vi "MHL Cases.vi"(8 "error in":errorcluster, 11 "Worker Base Class in":refnum<class "Worker Base Class.lvclass">) -> (0 "error out":errorcluster, 3 "Worker Base Class out":refnum<class "Worker Base Class.lvclass">)   [LabVIEW 2017, in "Worker Base Class.lvclass"]
doc: "The base class Message Handling Loop cases of a Worker's QMH."
uses:
  Worker Base Class.lvclass
  C:/Program Files (x86)/National Instruments/LabVIEW 2017/vi.lib/addons/_Workers/Library/Classes/Worker/Worker.lvclass
  <vilib>/addons/_Workers/Library/Classes/Worker/Worker.lvclass/Worker.ctl
  <vilib>/addons/_Workers/Library/Classes/Message/Message.lvclass/Message.ctl
  Initialization Data.ctl
  Response Cases.ctl
  Worker Base Class.lvclass/Worker Base Class.ctl
  rqp_Send message to Caller.ctl
  rqp_Send message to subWorkers.ctl
  <vilib>/addons/_Workers/Library/Classes/Worker/Worker.lvclass
  <vilib>/addons/_Workers/Library/Classes/Message/Message.lvclass
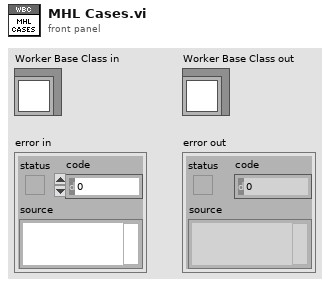
[diagram p1: front panel]
types:
  T1 = typedef "Workers.lvlib/Case Label.ctl" = string
  T2 = typedef "Worker Base Class.lvclass/Initialization Data.ctl" = cluster{"Response Cases":T3}
  T3 = typedef "Worker Base Class.lvclass/Response Cases.ctl" = cluster{"Placeholder - Can be deleted":string}
  T4 = typedef "Worker Base Class.lvclass/rqp_Send message to Caller.ctl" = cluster{"String":string}
  T5 = typedef "Worker Base Class.lvclass/rqp_Send message to subWorkers.ctl" = cluster{"String":string}
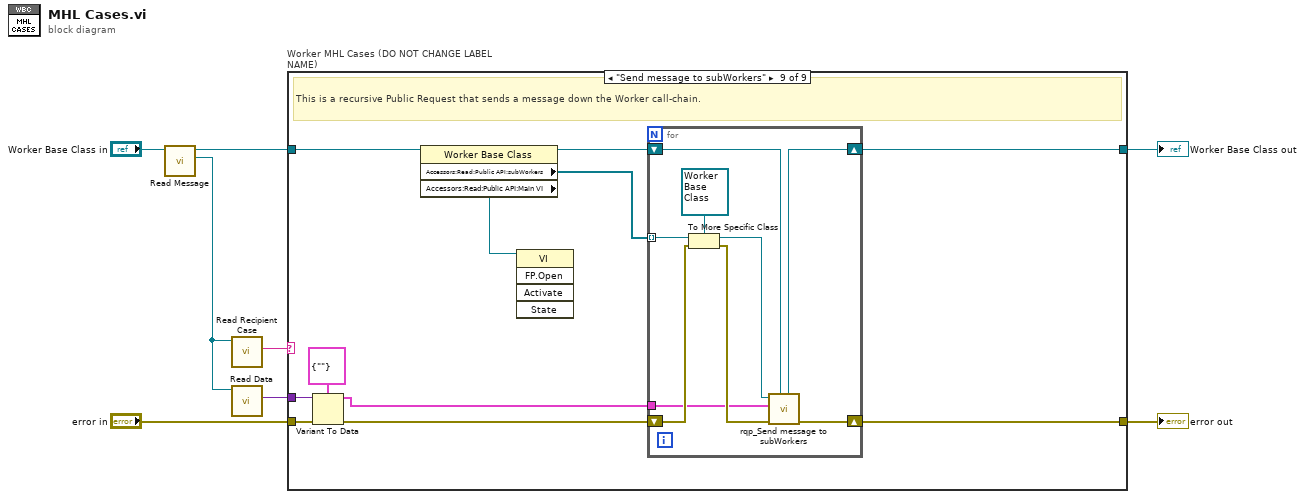
[diagram p0: block diagram]
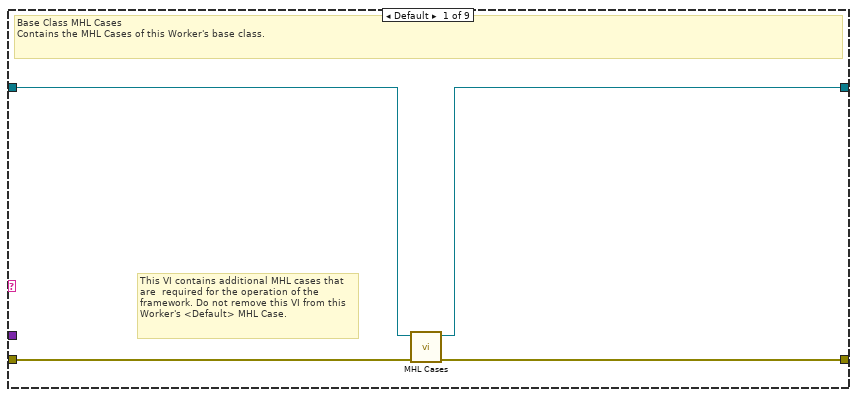
[diagram p2: hidden frame]
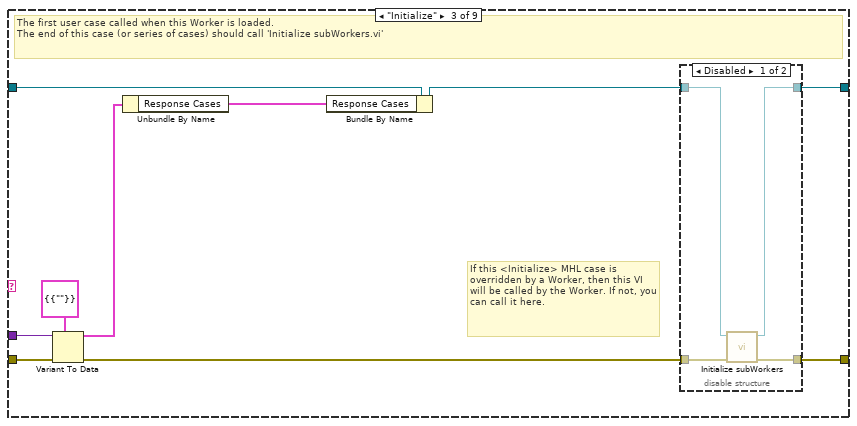
[diagram p4: hidden frame]
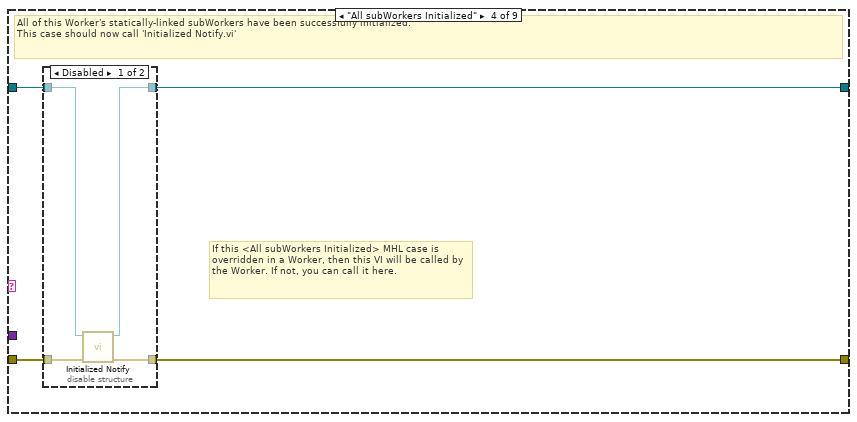
[diagram p6: hidden frame]
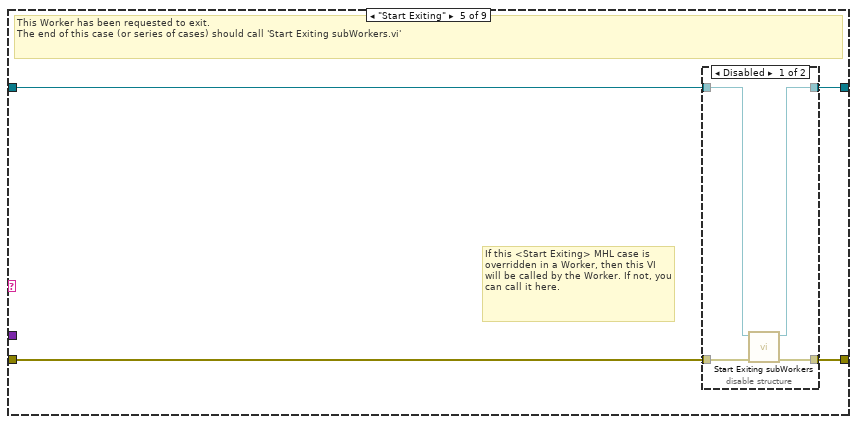
[diagram p8: hidden frame]
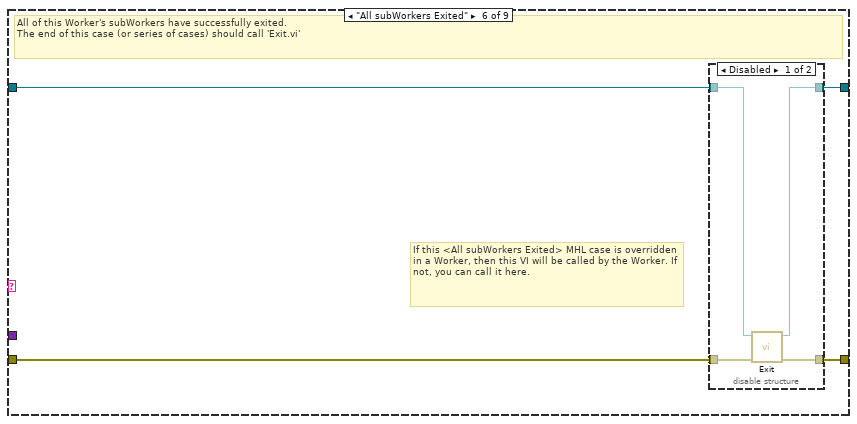
[diagram p10: hidden frame]
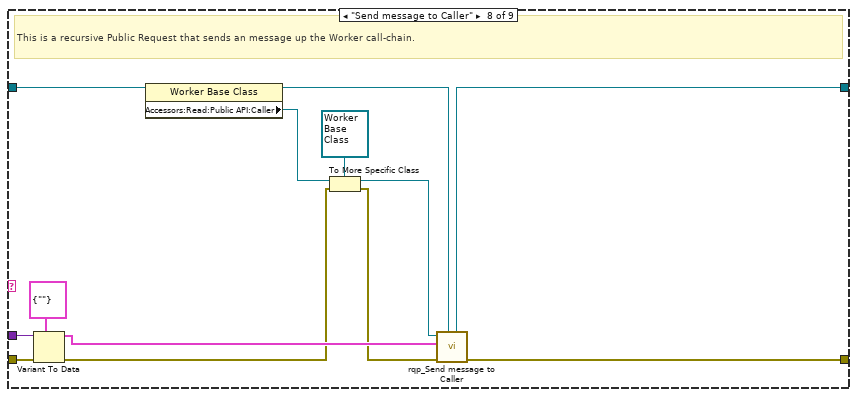
[diagram p13: hidden frame]
diagram:
  n1 = call <vilib>:"Read Message.vi"("Worker"="Worker Base Class in") -> ("Message"=w2:refnum<class "Message.lvclass">, "dup Worker out"=w8:refnum<class "Worker Base Class.lvclass">)  [unwired: 9 in]
  n2 = call <vilib>:"Read Recipient Case.vi"("Message"=w2) -> ("Recipient Case"=w7:T1)  [unwired: 9 in, 1 out]
  n3 = call <vilib>:"Read Data.vi"("Message"=w2) -> ("Data"=w1:variant)  [unwired: 9 in, 1 out]
  n4 = case "Worker MHL Cases (DO NOT CHANGE LABEL NAME)" shown="\"Send message to subWorkers\"" w7 {
    tunnel: [w12 w14 w17 w31 w42 w53 w62 w73 w82] -> w6
    tunnel: [w11 w13 w15 w33 w43 w51 w61 w71 w80] -> w5
    tunnel: "error in" -> [w10 w14 w24 w32 w41 w54 w62 w75 w86]
    tunnel: w8 -> [w9 w13 w23 w34 w44 w52 w61 w72 w81]
    tunnel: w1 -> [_ _ w22 _ _ _ _ w74 w83]
    frame Default {
      # "This VI contains additional MHL cases that are  required for the operation of the framework. Do not remove this VI from this Worker's <Default> MHL Case."
      # "Base Class MHL Cases\nContains the MHL Cases of this Worker's base class."
      n5 = call-parent "MHL Cases.vi"("error in"=w10, "Worker in"=w9) -> ("error out"=w12:errorcluster, "Worker out"=w11:refnum<class "Worker Base Class.lvclass">)  [unwired: 8 in]
    }
    frame "------------ FRAMEWORK CASES -----------" {
      # "Start of Workers Framework Cases"
    }
    frame "Initialize" {
      # "If this <Initialize> MHL case is overridden by a Worker, then this VI will be called by the Worker. If not, you can call it here."
      # "The first user case called when this Worker is loaded.\nThe end of this case (or series of cases) should call 'Initialize subWorkers.vi'"
      n6 = Variant To Data(error in=w24, type=T2 {"Response Cases"={"Placeholder - Can be deleted"=""}} ("Initialization Data"), Variant=w22) -> (data=w21:T2, error out=w18:errorcluster)
      n7 = Unbundle By Name(w21) -> ("Response Cases"=w20:T3)
      n8 = Bundle By Name(cluster=w23, "Response Cases"=w20) -> (w16:refnum<class "Worker Base Class.lvclass">)
      n9 = disable-structure shown="Disabled" {
        disable-tunnel: w18 -> [w28 w29]
        disable-tunnel: [w27 w29] -> w17
        disable-tunnel: w16 -> [w26 w30]
        disable-tunnel: [w25 w30] -> w15
        frame Disabled {
          n10 = call-dynamic "Initialize subWorkers.vi"("error in"=w28, "Worker"=w26) -> ("error out"=w27:errorcluster, "dup Worker out"=w25:refnum<class "Worker Base Class.lvclass">)  [unwired: 8 in]
        }
        frame Enabled {
        }
      }
    }
    frame "All subWorkers Initialized" {
      # "If this <All subWorkers Initialized> MHL case is overridden in a Worker, then this VI will be called by the Worker. If not, you can call it here."
      # "All of this Worker's statically-linked subWorkers have been successfully initialized.\nThis case should now call 'Initialized Notify.vi'"
      n11 = disable-structure shown="Disabled" {
        disable-tunnel: w34 -> [w38 w40]
        disable-tunnel: [w37 w40] -> w33
        disable-tunnel: w32 -> [w36 w39]
        disable-tunnel: [w35 w39] -> w31
        frame Disabled {
          n12 = call-dynamic "Initialized Notify.vi"("error in"=w36, "Worker"=w38) -> ("error out"=w35:errorcluster, "dup Worker out"=w37:refnum<class "Worker Base Class.lvclass">)  [unwired: 8 in]
        }
        frame Enabled {
        }
      }
    }
    frame "Start Exiting" {
      # "If this <Start Exiting> MHL case is overridden in a Worker, then this VI will be called by the Worker. If not, you can call it here."
      # "This Worker has been requested to exit. \nThe end of this case (or series of cases) should call 'Start Exiting subWorkers.vi'"
      n13 = disable-structure shown="Disabled" {
        disable-tunnel: w44 -> [w48 w50]
        disable-tunnel: [w47 w50] -> w43
        disable-tunnel: [w46 w49] -> w42
        disable-tunnel: w41 -> [w45 w49]
        frame Disabled {
          n14 = call-dynamic "Start Exiting subWorkers.vi"("error_in"=w45, "Worker"=w48) -> ("error out"=w46:errorcluster, "dup Worker out"=w47:refnum<class "Worker Base Class.lvclass">)  [unwired: 8 in]
        }
        frame Enabled {
        }
      }
    }
    frame "All subWorkers Exited" {
      # "If this <All subWorkers Exited> MHL case is overridden in a Worker, then this VI will be called by the Worker. If not, you can call it here."
      # "All of this Worker's subWorkers have successfully exited. \nThe end of this case (or series of cases) should call 'Exit.vi'"
      n15 = disable-structure shown="Disabled" {
        disable-tunnel: w54 -> [w58 w59]
        disable-tunnel: [w57 w59] -> w53
        disable-tunnel: w52 -> [w56 w60]
        disable-tunnel: [w55 w60] -> w51
        frame Disabled {
          n16 = call-dynamic "Exit.vi"("error_in"=w58, "Worker"=w56) -> ("error out"=w57:errorcluster, "dup Worker out"=w55:refnum<class "Worker Base Class.lvclass">)  [unwired: 8 in]
        }
        frame Enabled {
        }
      }
    }
    frame "------------- PUBLIC API CASES -------------" {
      # "Start of Workers Public API Cases"
    }
    frame "Send message to Caller" {
      # "This is a recursive Public Request that sends an message up the Worker call-chain."
      n17 = Variant To Data(error in=w75, type=T4 {"String"=""} ("Data"), Variant=w74) -> (data=w66:T4, error out=w65:errorcluster)
      n18 = property class="Worker Base Class"(reference=w72) -> (reference out=w70:refnum<class "Worker Base Class.lvclass">, "Accessors:Read:Public API:Caller"=w69:refnum<class "Worker.lvclass">)  [unwired: 1 in, 1 out]
      n19 = To More Specific Class(target class=refnum<class "Worker Base Class.lvclass"> refnum ("Worker Base Class"), reference=w69, error in=w65) -> (specific class reference=w68:refnum<class "Worker Base Class.lvclass">, error out=w64:errorcluster)
      n20 = call "rqp_Send message to Caller.vi"("Caller in"=w70, "error in"=w64, "Data in"=w66, "Worker Base Class in"=w68) -> ("error out"=w73:errorcluster, "dup Caller out"=w71:refnum<class "Worker Base Class.lvclass">)  [unwired: 5 in, 1 out]
    }
    frame "Send message to subWorkers" {
      # "This is a recursive Public Request that sends a message down the Worker call-chain."
      n21 = Variant To Data(error in=w86, type=T5 {"String"=""} ("Data"), Variant=w83) -> (data=w78:T5, error out=w85:errorcluster)
      n22 = property class="Worker Base Class"(reference=w81) -> (reference out=w79:refnum<class "Worker Base Class.lvclass">, "Accessors:Read:Public API:subWorkers"=w77:refnum<class "Worker.lvclass">[], "Accessors:Read:Public API:Main VI"=w76:refnum<vi>)  [unwired: 1 in, 1 out]
      n23 = invoke class="VI" method="FP.Open"(reference=w76) -> ()  [unwired: 4 in, 5 out]
      n24 = for {
        tunnel: w78 -> [w87]
        shift-right: [w95] -> w82
        shift-left: w85 -> [w89]
        shift-right: [w94] -> w80
        shift-left: w79 -> [w93]
        tunnel: w77 -> [w91] mode=indexing
        n25 = To More Specific Class(target class=refnum<class "Worker Base Class.lvclass"> refnum ("Worker Base Class"), reference=w91, error in=w89) -> (specific class reference=w90:refnum<class "Worker Base Class.lvclass">, error out=w88:errorcluster)
        n26 = call "rqp_Send message to subWorkers.vi"("Caller in"=w93, "error in"=w88, "Data in"=w87, "Worker Base Class in"=w90) -> ("error out"=w95:errorcluster, "dup Caller out"=w94:refnum<class "Worker Base Class.lvclass">)  [unwired: 5 in, 1 out]
      }
    }
  }
  "Worker Base Class out" <- w5
  "error out" <- w6
